vi "Update Task Infos.vi"(8 "error in (no error)":errorcluster, 10 "Task":i32, 11 "Task Setting Editor in":refnum<class "Task Setting Editor.lvclass">) -> (0 "error out":errorcluster, 3 "Task Setting Editor out":refnum<class "Task Setting Editor.lvclass">)   [LabVIEW 2017, in "Task Setting Editor.lvlib" / "Task Setting Editor.lvclass"]
uses:
  Task Setting Editor.lvclass
  Task Setting Editor.lvclass/Task Setting Editor.ctl
  BuildWorker/Classes/Task/Task.lvclass/Task.ctl
  BuildWorker/Classes/Task/Get Name.vi
  BuildWorker/Classes/Task/Get Target.vi
  BuildWorker/Classes/Task/Read BuildSpec Type.vi
  BuildWorker/Classes/Task/Get BuildSpec Name.vi
  BuildWorker/Classes/Task/Get ProjectPath.vi
  BuildWorker/Classes/Task/Read Worker.vi
  BuildWorker/Classes/Task/Read Display Name.vi
  BuildWorker/Classes/Task/Get ProjectName.vi
  BuildWorker/Classes/Task/Get Status String.vi
  BuildWorker/Classes/Task/Task.lvclass
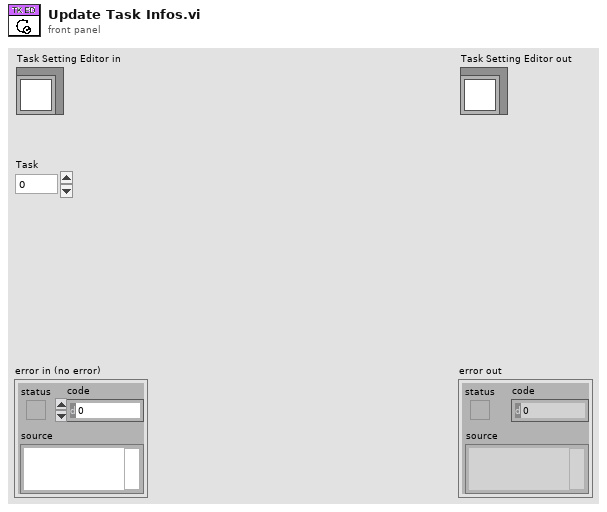
[diagram p1: front panel]
types:
  T1 = cluster{"Display Name":refnum<vi>, "Worker":refnum<vi>}
  T2 = cluster{"Name":refnum<vi>, "ProjectName":refnum<vi>, "Target":refnum<vi>, "BuildSpec Type":refnum<vi>, "BuildSpec Name":refnum<vi>, "ProjectPath":refnum<vi>, "Status string":refnum<vi>}
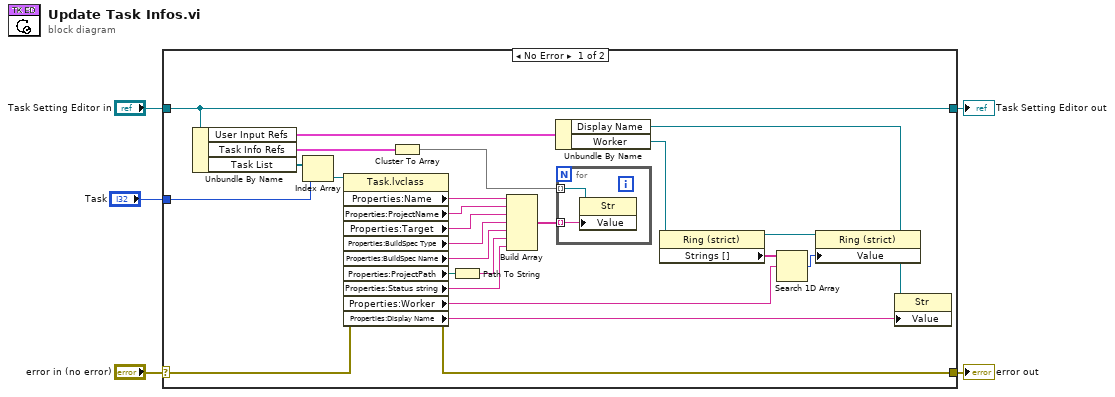
[diagram p0: block diagram]
diagram:
  n1 = case shown="No Error" "error in (no error)" {
    selector: "error in (no error)" -> [w26 w34]
    tunnel: [w25 w34] -> w4
    tunnel: [w30 w33] -> w2
    tunnel: "Task Setting Editor in" -> [w30 w33]
    tunnel: "Task" -> [w28 _]
    frame No Error {
      n2 = Unbundle By Name(w30) -> ("User Input Refs"=w16:T1, "Task Info Refs"=w12:T2, "Task List"=w29:refnum<class "Task.lvclass">[])
      n3 = Index Array(array=w29, index=w28) -> (element=w27:refnum<class "Task.lvclass">)
      n4 = property class="Task.lvclass"(reference=w27, error in=w26) -> (error out=w25:errorcluster, "Properties:Name"=w24:string, "Properties:ProjectName"=w23:string, "Properties:Target"=w11:string, "Properties:BuildSpec Type"=w22:string, "Properties:BuildSpec Name"=w21:string, "Properties:ProjectPath"=w20:path, "Properties:Status string"=w19:string, "Properties:Worker"=w8:string, "Properties:Display Name"=w13:string)  [unwired: 1 out]
      n5 = Cluster To Array(cluster=w12) -> (array=w18:refnum<vi>[])
      n6 = Path To String(path=w20) -> (string=w10:string)
      n7 = Build Array(w24, w23, w11, w22, w21, w10, w19) -> (w17:string[])
      n8 = Unbundle By Name(w16) -> ("Display Name"=w14:refnum<vi>, "Worker"=w15:refnum<vi>)
      n9 = for {
        tunnel: w18 -> [w32] mode=indexing
        tunnel: w17 -> [w31] mode=indexing
        n10 = property class="Str"(reference=w32, "Value"=w31) -> ()  [unwired: 1 in, 2 out]
      }
      n11 = property class="Ring (strict)"(reference=w15) -> (reference out=w7:refnum<vi>, "Strings []"=w9:string[])  [unwired: 1 in, 1 out]
      n12 = Search 1D Array(1D array=w9, element=w8) -> (index of element=w6:i32)  [unwired: 1 in]
      n13 = property class="Ring (strict)"(reference=w7, "Value"=w6) -> ()  [unwired: 1 in, 2 out]
      n14 = property class="Str"(reference=w14, "Value"=w13) -> ()  [unwired: 1 in, 2 out]
    }
    frame Error {
    }
  }
  "error out" <- w4
  "Task Setting Editor out" <- w2
